vi "GeoFonu_v1.6.vi"() -> ()   [LabVIEW 2014]
uses:
  <vilib>/Instr/_visa.llb/VISA Set IO Buffer Mask.ctl
  <vilib>/Instr/_visa.llb/VISA Flush IO Buffer Mask.ctl
  <vilib>/Instr/_visa.llb/VISA Configure Serial Port (Instr).vi
panel:
  out "ReceivedBytes":i32(graph)
  out "Real time":timestamp
  out "Sensor3 x 5":i32[](graph)=[361, 364, 361, 361, 360, 361, 362, 365, 364, 360, 364, 365, 361, 363, 364, 364, 361, 361, 364, 361, 364, 365, 362, 363, 364, 360, 362, 361, 364, 362, 362, 364, 363, 363, 365, 361, 363, 362, 363, 361, 361, 364, 364, 361, 361, 362, 361, 363, 361, 363, 363, 359, 362, 360, 361, 360, 362, 360, 363, 361, 361, 361, 361, 364, 361, 360, 359, 361, 364, 368, 366, 363, 364, 361, 360, 363, 361, 364, 359, 364, 364, 363, 361, 362, 363, 361, 364, 363, 362, 364, 361, 364, 363, 364, 363, 366, 360, 361, 360, 362, 362, 361, 363, 361, 366, 362, 361, 363, 362, 364, 364, 362, 362, 364, 362, 360, 364, 358, 364, 365, 361, 362, 364, 360, 361, 361, 365, 363, 365, 362, 364, 361, 361, 362, 364, 365, 361, 364, 362, 359, 359, 359, 361, 362, 361, 361, 360, 362, 364, 361, 360, 364, 361, 359, 364, 362, 364, 361, 365, 361, 363, 359, 362, 360, 361, 363, 361, 361, 362, 361, 361, 364, 363, 363, 362, 361, 361, 363, 359, 363, 362, 360, 363, 362, 362, 361, 362, 363, 363, 362, 358, 359, 363, 362, 362, 362, 364, 363, 364, 367, 362, 362, 362, 363, 364, 362, 363, 365, 362, 362, 362, 363, 362, 363, 362, 365, 360, 357, 362, 362, 362, 359, 363, 362, 363, 363, 359, 361, 359, 364, 360, 360, 367, 358, 360, 364, 367, 362, 362, 361, 362, 362, 364, 361, 361, 362, 365, 360, 364, 364, 361, 362, 360, 359, 364, 363, 364, 361, 362, 359, 362, 362, 358, 360, 364, 364, 359, 362, 363, 363, 361, 365, 363, 361, 357, 361, 364, 362, 364, 361, 365, 362, 361, 361, 362, 360, 363, 360, 362, 363, 363, 361, 359, 362, 363, 362, 364, 360, 362, 365, 359, 361, 365, 362, 364, 362, 362, 363, 363, 361, 362, 364, 361, 363, 361, 361, 364, 362, 362, 360, 362, 362, 360, 363, 364, 360, 360, 363, 362, 361, 360, 360, 361, 360, 361, 361, 365, 358, 361, 363, 362, 364, 361, 364, 362, 361, 361, 368, 360, 362, 360, 360, 363, 359, 367, 365, 361, 362, 361, 360, 367, 362, 362, 362, 363, 362, 362, 363, 362, 364, 361, 365, 360, 363, 360, 364, 358, 360, 362, 364, 361, 362, 363, 358, 364, 363, 364, 364, 363, 365, 362, 361, 365, 362, 360, 362, 361, 364, 363, 361, 362, 367, 362, 362, 361, 364, 366, 361, 362, 362, 359, 362, 362, 365, 362, 363, 363, 364, 362, 364, 362, 365, 361, 362, 361, 362, 362, 362, 363, 359, 362, 365, 362, 361, 368, 360, 363, 361, 365, 364, 362, 364, 364, 362, 362, 363, 362, 362, 362, 361, 359, 365, 361, 362, 362, 362, 362, 367, 362, 362, 360, 362, 362, 361, 362, 363, 362, 363, 363, 363, 362, 362, 359, 362, 362, 362, 361, 362, 362, 362, 360, 360, 360, 363, 360, 363, 364, 364, 359, 360, 360, 365, 365, 363, 362, 362, 364, 363, 364, 367, 360, 362]
  out "Sensor2 x10":i32[](graph)=[224, 220, 225, 225, 222, 223, 225, 223, 224, 225, 223, 225, 225, 226, 224, 225, 222, 222, 223, 224, 225, 224, 221, 225, 226, 225, 223, 223, 224, 222, 223, 227, 225, 224, 224, 224, 220, 224, 225, 221, 223, 225, 225, 223, 221, 225, 224, 224, 223, 222, 224, 223, 226, 225, 224, 224, 223, 222, 221, 224, 224, 221, 222, 224, 221, 225, 225, 225, 225, 227, 223, 228, 223, 226, 223, 225, 223, 223, 224, 225, 226, 226, 227, 222, 223, 221, 224, 223, 225, 224, 223, 223, 224, 226, 227, 224, 222, 223, 226, 225, 224, 224, 220, 221, 220, 225, 224, 226, 224, 223, 223, 224, 221, 223, 221, 225, 224, 224, 225, 228, 224, 224, 223, 225, 225, 223, 224, 221, 223, 223, 225, 224, 221, 224, 223, 225, 223, 223, 225, 222, 225, 224, 223, 223, 225, 225, 223, 223, 223, 223, 223, 224, 225, 224, 225, 223, 225, 224, 225, 223, 222, 223, 223, 222, 222, 224, 221, 223, 221, 223, 224, 225, 225, 224, 223, 222, 225, 223, 222, 226, 225, 225, 224, 223, 220, 222, 225, 221, 224, 223, 227, 223, 222, 226, 226, 223, 222, 226, 221, 225, 224, 224, 224, 226, 224, 222, 224, 224, 223, 224, 227, 226, 226, 226, 222, 222, 222, 225, 223, 226, 225, 222, 226, 224, 225, 225, 224, 225, 223, 224, 222, 223, 224, 224, 228, 222, 226, 221, 224, 226, 224, 224, 222, 224, 224, 222, 224, 225, 224, 225, 223, 223, 221, 224, 225, 226, 225, 222, 224, 224, 226, 226, 225, 225, 227, 224, 222, 223, 222, 224, 223, 221, 224, 225, 223, 225, 224, 223, 227, 224, 225, 224, 225, 223, 223, 225, 221, 222, 224, 224, 225, 222, 224, 222, 224, 223, 224, 225, 224, 222, 225, 223, 225, 223, 221, 224, 223, 224, 224, 222, 225, 225, 224, 226, 222, 224, 224, 225, 223, 225, 225, 226, 225, 224, 224, 223, 223, 223, 223, 222, 224, 222, 223, 227, 224, 224, 225, 226, 226, 224, 223, 224, 223, 225, 227, 223, 224, 224, 225, 224, 224, 224, 224, 224, 223, 226, 224, 221, 226, 226, 226, 224, 226, 227, 226, 226, 223, 226, 224, 225, 224, 225, 226, 225, 222, 223, 227, 224, 224, 224, 224, 226, 222, 224, 225, 222, 224, 226, 226, 228, 226, 224, 224, 221, 222, 224, 223, 224, 224, 224, 224, 226, 225, 224, 221, 224, 227, 222, 225, 224, 225, 225, 223, 222, 223, 224, 224, 224, 222, 224, 222, 226, 222, 227, 225, 222, 224, 224, 221, 224, 225, 226, 223, 225, 224, 222, 224, 224, 223, 226, 225, 224, 224, 224, 223, 225, 224, 224, 224, 225, 223, 224, 222, 224, 226, 223, 224, 224, 223, 226, 227, 224, 224, 225, 227, 223, 226, 228, 226, 226, 221, 225, 224, 226, 226, 224, 224, 226, 226, 227, 226, 224, 225, 223, 224, 224, 224, 225, 223, 226, 223, 227, 223, 228, 226, 228, 225, 227, 225, 223, 224, 225]
  out "Sensor1 x 1":i32[](graph)=[259, 257, 260, 259, 256, 260, 261, 261, 259, 259, 256, 260, 259, 260, 256, 258, 258, 260, 260, 259, 259, 259, 261, 259, 261, 258, 259, 260, 261, 258, 257, 257, 261, 258, 259, 260, 259, 259, 259, 260, 261, 260, 260, 262, 259, 259, 258, 259, 261, 259, 261, 257, 260, 260, 257, 258, 262, 261, 261, 261, 258, 259, 257, 261, 259, 259, 262, 258, 259, 259, 260, 260, 259, 259, 260, 263, 262, 259, 260, 263, 262, 257, 258, 262, 261, 259, 261, 259, 261, 260, 259, 263, 259, 261, 260, 258, 263, 259, 259, 260, 260, 256, 258, 259, 264, 259, 259, 260, 259, 258, 259, 262, 262, 264, 260, 264, 260, 262, 261, 261, 262, 259, 261, 261, 261, 260, 259, 261, 260, 259, 260, 261, 258, 261, 260, 261, 261, 263, 260, 261, 260, 259, 258, 261, 258, 261, 261, 259, 259, 262, 260, 259, 262, 259, 260, 258, 261, 259, 260, 261, 261, 259, 259, 260, 260, 259, 259, 261, 257, 262, 261, 262, 259, 259, 257, 260, 260, 260, 260, 259, 261, 260, 259, 259, 259, 262, 260, 261, 263, 259, 261, 265, 260, 260, 260, 260, 260, 260, 260, 258, 261, 259, 261, 260, 262, 260, 262, 262, 260, 264, 260, 260, 260, 261, 263, 264, 260, 261, 260, 264, 260, 264, 262, 260, 261, 262, 260, 260, 260, 260, 261, 260, 261, 260, 263, 259, 260, 260, 261, 259, 260, 260, 264, 260, 262, 260, 257, 256, 262, 260, 258, 261, 259, 260, 262, 263, 258, 258, 263, 260, 262, 263, 260, 262, 256, 260, 260, 260, 262, 262, 260, 260, 263, 259, 262, 266, 259, 260, 260, 263, 260, 260, 261, 260, 262, 260, 262, 258, 259, 261, 262, 260, 258, 260, 259, 260, 263, 263, 260, 260, 260, 261, 262, 261, 262, 263, 262, 261, 260, 263, 260, 262, 259, 260, 258, 259, 260, 260, 260, 261, 260, 261, 258, 262, 262, 260, 262, 259, 262, 260, 260, 263, 260, 259, 258, 262, 264, 261, 258, 259, 262, 260, 260, 261, 259, 260, 262, 260, 263, 260, 261, 263, 263, 264, 262, 260, 264, 260, 257, 260, 261, 262, 261, 260, 260, 262, 259, 261, 261, 263, 259, 260, 261, 259, 260, 258, 260, 260, 259, 261, 260, 262, 259, 260, 261, 260, 261, 262, 262, 261, 261, 262, 262, 260, 263, 260, 261, 262, 259, 261, 262, 263, 263, 263, 262, 262, 262, 264, 260, 257, 260, 262, 261, 262, 258, 262, 261, 260, 260, 258, 258, 262, 260, 260, 260, 262, 261, 262, 265, 260, 263, 258, 261, 261, 260, 263, 258, 263, 261, 259, 260, 258, 257, 262, 259, 264, 261, 262, 263, 261, 263, 262, 258, 260, 260, 261, 259, 261, 263, 262, 259, 260, 260, 258, 262, 263, 260, 260, 260, 261, 259, 263, 259, 258, 262, 260, 259, 264, 258, 264, 260, 262, 261, 261, 262, 260, 260, 262, 259, 258, 260, 260, 260, 260, 258, 265, 261, 261, 264, 265, 262, 263]
  in  "milliseconds to wait":u32=500
  in  "stop":bool
  in  "VISA resource name":refnum<visa-resource-name>
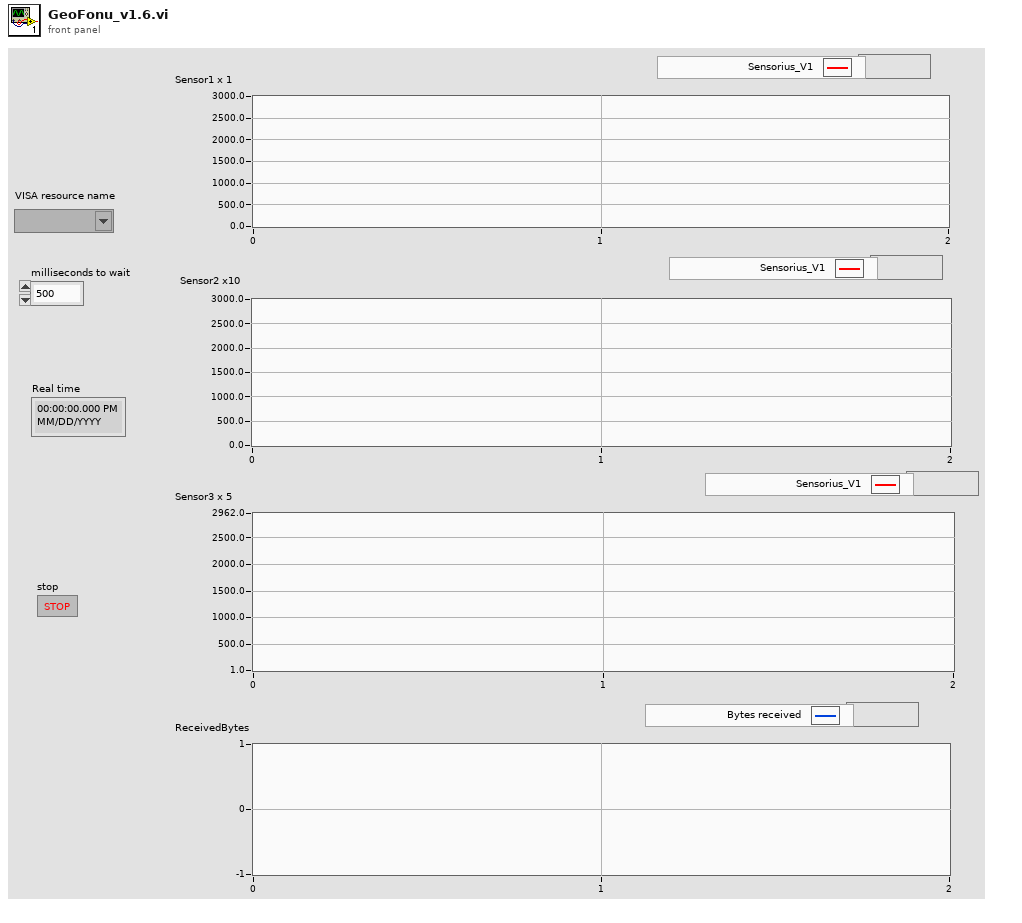
[diagram p1: front panel]
types:
  T1 = typedef "VISA Set IO Buffer Mask.ctl" = u16
  T2 = typedef "VISA Flush IO Buffer Mask.ctl" = u16
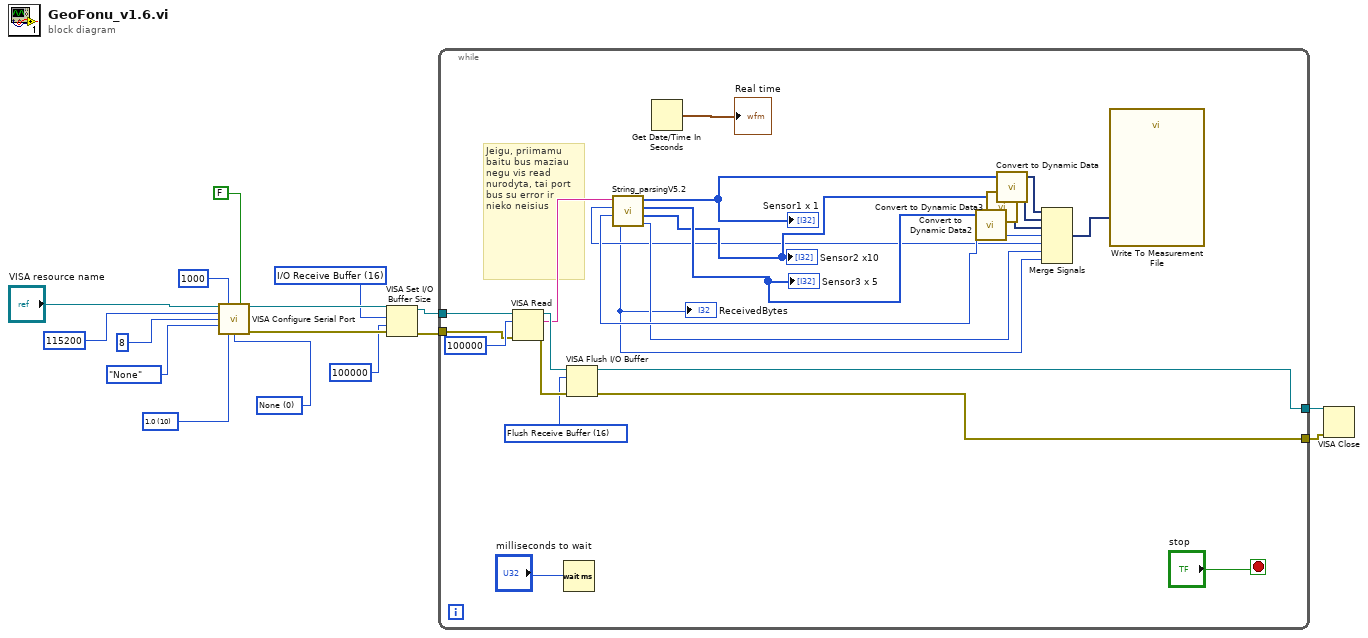
[diagram p0: block diagram]
diagram:
  w6 = T1 16 items=["I/O Receive Buffer"=16, "I/O Transmit Buffer"=32, "I/O Receive and Transmit Buffer"=48] ("Mask")
  w12 = u16 0 items=["None", "XON/XOFF", "RTS/CTS", "XON/XOFF & RTS/CTS", "DTR/DSR", "XON/XOFF & DTR/DSR"] ("flow control (0:none)")
  w13 = u16 10 items=["1.0"=10, "1.5"=15, "2.0"=20] ("stop bits (10: 1 bit)")
  n1 = call-poly "VISA Configure Serial Port"("VISA resource name"="VISA resource name", "timeout (10sec)"=u32 1000, "Enable Termination\nChar (T)"=FALSE ("Enable Termination\nChar (T)"), "baud rate (9600)"=u32 115200, "data bits (8)"=u16 8, "parity (0:none)"=enum16{"None", "Odd", "Even", "Mark", "Space"}."None", "stop bits (10: 1 bit)"=w13, "flow control (0:none)"=w12) -> ("VISA resource name out"=w8:refnum<visa-resource-name>, "error out"=w9:errorcluster)  [unwired: 6 in]
  n2 = VISA Set I/O Buffer Size(VISA resource name=w8, mask (16)=w6, size (4096)=u32 100000, error in (no error)=w9) -> (VISA resource name out=w3:refnum<visa-resource-name>, error out=w5:errorcluster)
  n3 = while {
    tunnel: w3 -> [w39]
    tunnel: w5 -> [w36]
    tunnel: [w31] -> w2
    tunnel: [w30] -> w1
    stop <- "stop" stop-if-true
    w33 = T2 16 items=["Flush Receive Buffer"=16, "Write Transmit Buffer to Device"=32, "Flush Receive Buffer (No I/O)"=64, "Flush Transmit Buffer"=128] ("Mask")
    # "Jeigu, priimamu baitu bus maziau negu vis read nurodyta, tai port bus su error ir nieko neisius"
    n4 = VISA Read(VISA resource name=w39, byte count=u32 100000, error in (no error)=w36) -> (VISA resource name out=w35:refnum<visa-resource-name>, read buffer=w25:string, error out=w34:errorcluster)  [unwired: 1 out]
    n5 = Wait (ms)(milliseconds to wait="milliseconds to wait") -> ()  [unwired: 1 out]
    n6 = VISA Flush I/O Buffer(VISA resource name=w35, mask (16)=w33, error in (no error)=w34) -> (VISA resource name out=w31:refnum<visa-resource-name>, error out=w30:errorcluster)
    n7 = call "String_parsingV5.2.vi"("input string"=w25) -> ("hour"=w20:i32, "V2"=w22:i32[], "V3"=w23:i32[], "V1"=w24:i32[], "size(s)"=w17:i32, "sekundes"=w21:i32, "minute"=w18:i32)
    "Sensor1 x 1" <- w24
    "Sensor2 x10" <- w22
    "Sensor3 x 5" <- w23
    "ReceivedBytes" <- w17
    n8 = Get Date/Time In Seconds() -> (seconds since 1Jan1904=→"Real time":timestamp)
    n9 = call "Convert to Dynamic Data2"("Array"=w23) -> ("Dynamic Data Type"=w27:dynamicdata)  [unwired: 3 in]
    n10 = call "Convert to Dynamic Data3"("Array"=w22) -> ("Dynamic Data Type"=w26:dynamicdata)  [unwired: 3 in]
    n11 = call "Convert to Dynamic Data"("Array"=w24) -> ("Dynamic Data Type"=w29:dynamicdata)  [unwired: 3 in]
    n12 = Merge Signals(w29, w26, w27, w21, w18, w20, w17) -> (w28:dynamicdata)
    n13 = call "Write To Measurement File"("Signals"=w28) -> ()  [unwired: 16 in, 3 out]
  }
  n14 = VISA Close(VISA resource name=w2, error in (no error)=w1) -> ()  [unwired: 1 out]
